vi "Emit.vi"(6 "inparameter":variant, 8 "error in (no error)":errorcluster, 9 "parameter":variant, 10 "function":string, 11 "output_actor in":refnum<class "Output Actor.lvclass">) -> (0 "error out":errorcluster, 3 "output_actor out":refnum<class "Output Actor.lvclass">)   [LabVIEW 2015, in "Output Actor.lvclass"]
uses:
  Output Actor.lvclass
  Output Actor.lvclass/Output Actor.ctl
  Output/Output.lvclass
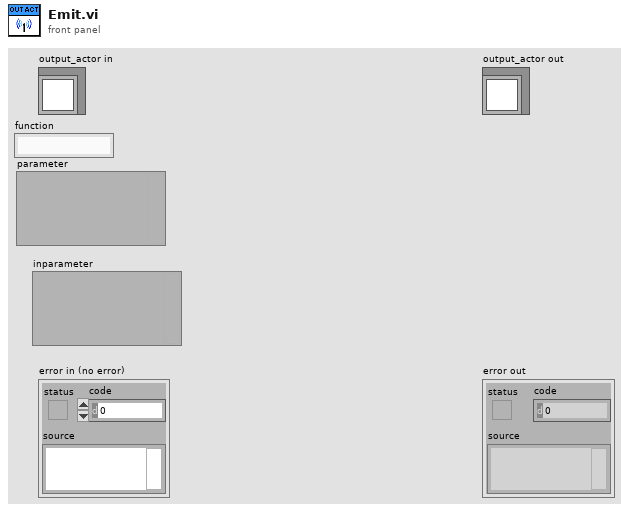
[diagram p1: front panel]
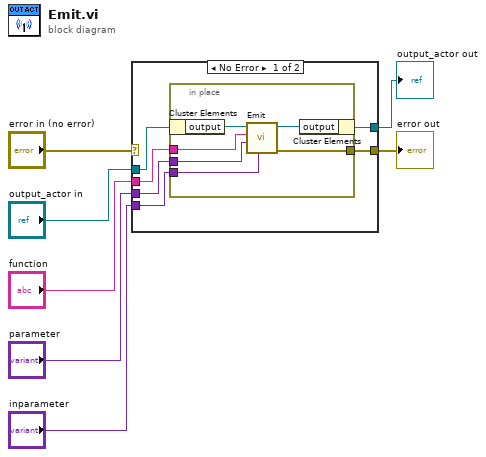
[diagram p0: block diagram]
diagram:
  n1 = case shown="No Error" "error in (no error)" {
    selector: "error in (no error)" -> [_ w21]
    tunnel: [w9 w21] -> w6
    tunnel: [w8 w20] -> w4
    tunnel: "output_actor in" -> [w13 w20]
    tunnel: "function" -> [w12 _]
    tunnel: "parameter" -> [w11 _]
    tunnel: "inparameter" -> [w10 _]
    frame No Error {
      n2 = in-place {
        in-place-border: w12 -> [w17]
        in-place-border: w11 -> [w16]
        in-place-border: w10 -> [w15]
        in-place-border: [w14] -> w9
        n3 = in-place-cluster #1(w13) -> ("output"=w19:refnum<class "Output.lvclass">)
        n4 = call "Emit.vi"("inparameter"=w15, "parameter"=w16, "function"=w17, "output in"=w19) -> ("error out"=w14:errorcluster, "output out"=w18:refnum<class "Output.lvclass">)  [unwired: 6 in]
        n5 = in-place-cluster #1("output"=w18) -> (w8:refnum<class "Output Actor.lvclass">)
      }
    }
    frame Error {
    }
  }
  "error out" <- w6
  "output_actor out" <- w4
